vi "test_sftp.vi"(5 "Close":bool, 7 "Connection Info.":T1={"Remote"="", "Username"="", "Port (22)"=22}, 8 "error in (no error)":errorcluster, 9 "Operation":enum16{"DownLoad", "file_list"}(ring), 10 "Local folder":path=path "C:/Working Folder/ssh.git", 11 "Remote File Path":string="/home/greg/Documents/Test.txt") -> (0 "error out":errorcluster, 2 "folder&file List":string[](array[string]))   [LabVIEW 2022 SP3]
uses:
  SFTP Library/Connection Info..cluster.ctl
  SFTP Library/Password..cluster.ctl
  68e57ec1-ca4e-4698-972b-b39e96289c7d.vi
  <vilib>/Utility/error.llb/Trim Whitespace One-Sided.vi
  SFTP Library/connect_password.vi
  <vilib>/Comparison/Less/Less Functor/Less Functor.lvclass
  SFTP Library/LabSFTP.lvlib
panel:
  out "folder&file List":string
  out "Method Response":string
  out "isSftpConnected":bool
  in  "Output":string
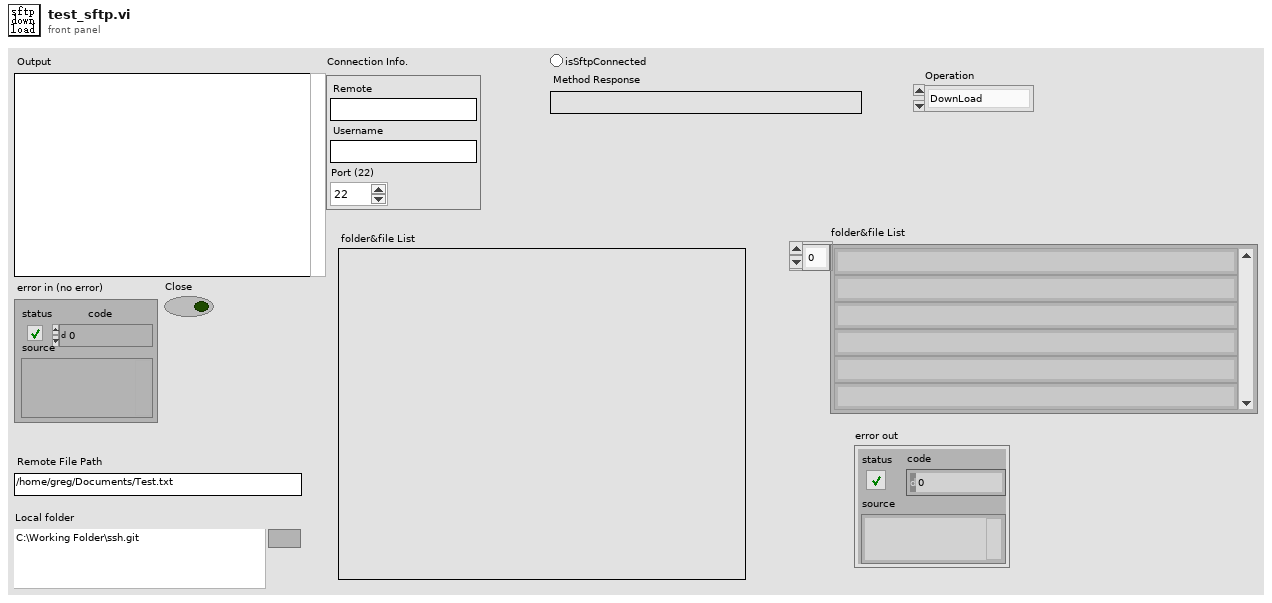
[diagram p1: front panel]
types:
  T1 = typedef "LabSFTP.lvlib/Connection Info..cluster.ctl" = cluster{"Remote":string, "Username":string, "Port (22)":i32}
  T2 = typedef "LabSFTP.lvlib/Password..cluster.ctl" = cluster{"Password":string}
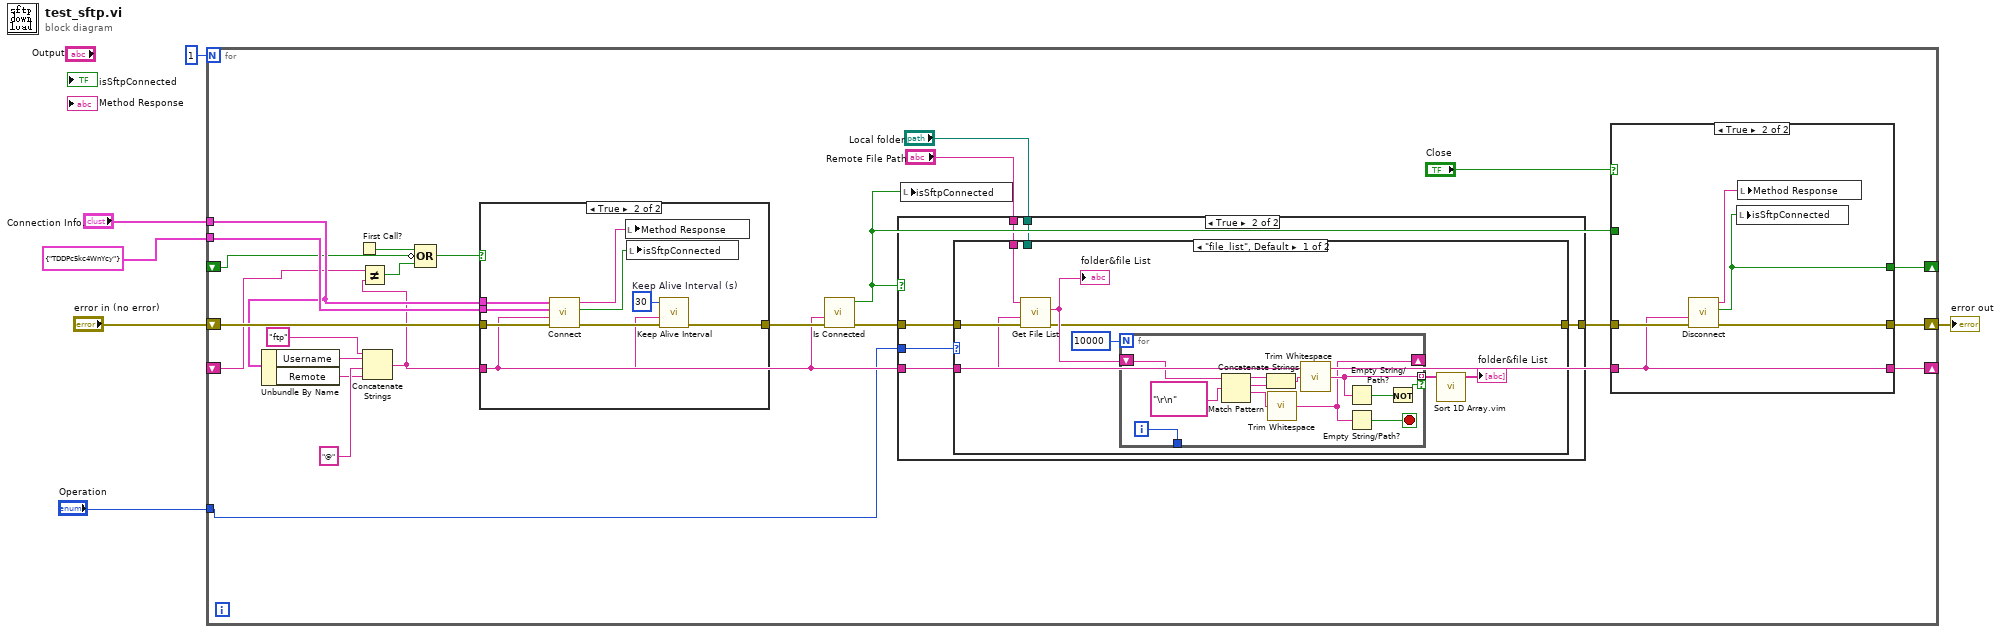
[diagram p0: block diagram]
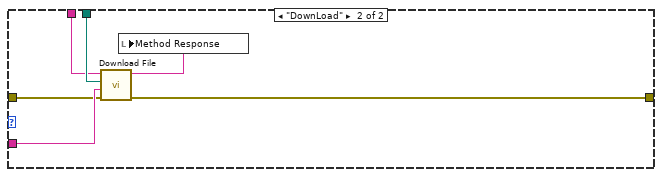
[diagram p5: hidden frame]
diagram:
  n1 = for {
    N: 1 -> [_]
    tunnel: T2 {"Password"="TDDPc5kc4WnYcy"} ("Password") -> [w25]
    tunnel: "Connection Info." -> [w19]
    shift-right: [w17] -> w2
    shift-left: "error in (no error)" -> [w24]
    shift-right: [w16] -> _
    shift-left: _ -> [w12]
    shift-right: [w14] -> _
    shift-left: _ -> [w11]
    tunnel: "Operation" -> [w7]
    n2 = Unbundle By Name(w19) -> ("Username"=w21:string, "Remote"=w22:string)
    n3 = First Call?() -> (First Call?: T/F=w13:bool)
    n4 = Concatenate Strings("ftp" ("string"), w21, "@" ("string"), w22) -> (w10:string)
    n5 = Not Equal?(x=w11, y=w10) -> (x != y?=w9:bool)
    n6 = Compound Arithmetic op=OR(w13, invert w12, w9) -> (w8:bool)
    n7 = case shown="True" w8 {
      tunnel: [w31 w38] -> w27
      tunnel: w25 -> [_ w35]
      tunnel: w24 -> [w31 w34]
      tunnel: w19 -> [_ w33]
      tunnel: w10 -> [_ w32]
      frame False {
      }
      frame True {
        w36 = 30  # Keep Alive Interval (s)
        n8 = call-poly "Connect.vi"("error in (no error)"=w34, "Connection Name"=w32, "Password"=w35, "Connection Info."=w33) -> ("error out"=w37:errorcluster, "isSftpConnected"=w40:bool, "Return String"=w39:string)  [unwired: 5 in]
        n9 = local write "Method Response"(w39) -> ()
        n10 = local write "isSftpConnected"(w40) -> ()
        n11 = call "Keep Alive Interval.vi"("error in (no error)"=w37, "Connection Name"=w32, "Keep Alive Interval (s)"=w36) -> ("error out"=w38:errorcluster)  [unwired: 8 in]
      }
    }
    n12 = call "Is Connected.vi"("error in (no error)"=w27, "Connection Name"=w10) -> ("error out"=w30:errorcluster, "isSshConnected"=w15:bool)  [unwired: 8 in]
    n13 = case shown="True" w15 {
      tunnel: w30 -> [w49 w51]
      tunnel: [w49 w55] -> w29
      tunnel: "Remote File Path" -> [_ w52]
      tunnel: "Local folder" -> [_ w54]
      tunnel: w10 -> [_ w53]
      tunnel: w7 -> [_ w50]
      frame False {
      }
      frame True {
        n14 = case shown="\"file_list\", Default" w50 {
          tunnel: [w56 w81] -> w55
          tunnel: w54 -> [_ w79]
          tunnel: w53 -> [w62 w78]
          tunnel: w52 -> [w61 w77]
          tunnel: w51 -> [w63 w76]
          frame "file_list", Default {
            n15 = call "Get File List.vi"("error in (no error)"=w63, "Connection Name"=w62, "Remote Path"=w61) -> ("error out"=w56:errorcluster, "File List"=w57:string)  [unwired: 6 in, 1 out]
            "folder&file List" <- w57
            n16 = for {
              N: 10000 -> [_]
              tunnel: [w72] -> w59 mode=indexing if=w70
              shift-right: [w66] -> _
              shift-left: w57 -> [w75]
              tunnel: [w64] -> _
              i -> [w64]
              stop <- w65 stop-if-true
              n17 = Match Pattern(string=w75, regular expression="\r\n") -> (before substring=w73:string, match substring=w68:string, after substring=w67:string)  [unwired: 1 in, 1 out]
              n18 = Concatenate Strings(w73, w68) -> (w69:string)
              n19 = call <vilib>:"Trim Whitespace.vi"("string"=w67) -> ("trimmed string"=w66:string)  [unwired: 1 in]
              n20 = call <vilib>:"Trim Whitespace.vi"("string"=w69) -> ("trimmed string"=w72:string)  [unwired: 1 in]
              n21 = Empty String/Path?(string/path=w72) -> (empty?=w71:bool)
              n22 = Empty String/Path?(string/path=w66) -> (empty?=w65:bool)
              n23 = Not(x=w71) -> (.not. x?=w70:bool)
            }
            n24 = call "Sort 1D Array.vim"("unsorted array"=w59) -> ("sorted array"=→"folder&file List":string[])  [unwired: 10 in]
          }
          frame "DownLoad" {
            n25 = call "Download File.vi"("error in (no error)"=w76, "Connection Name"=w78, "Local File Path"=w79, "Remote File Path"=w77) -> ("error out"=w81:errorcluster, "Return String"=w80:string)  [unwired: 6 in]
            n26 = local write "Method Response"(w80) -> ()
          }
        }
      }
    }
    n27 = local write "isSftpConnected"(w15) -> ()
    n28 = case shown="True" "Close" {
      tunnel: w29 -> [w43 w47]
      tunnel: w10 -> [w41 w44]
      tunnel: [w43 w46] -> w17
      tunnel: [w42 w45] -> w16
      tunnel: w15 -> [w42 _]
      tunnel: [w41 w44] -> w14
      frame False {
      }
      frame True {
        n29 = call "Disconnect.vi"("error in (no error)"=w47, "Connection Name"=w44) -> ("error out"=w46:errorcluster, "isSshConnected"=w45:bool, "Return String"=w48:string)  [unwired: 7 in]
        n30 = local write "isSftpConnected"(w45) -> ()
        n31 = local write "Method Response"(w48) -> ()
      }
    }
  }
  "error out" <- w2
